vi "SwapInstanceVIUnusedName2 40.vi"(6 "Bindata & descr in":T1, 7 "type":i16, 8 "error in (no error)":errorcluster, 9 "dims":u8=3 min=1 max=3, 11 "kwarg_name":string="testarg") -> (0 "error out":errorcluster, 1 "Array 3D":i16[][][](array[numeric]), 2 "Array 2D":i16[][](array[numeric]), 3 "Array 1D":i16[](array[numeric]), 4 "Bindata & descr out":T1, 5 "bindata":u8[](array[numeric]))   [LabVIEW 2018]
uses:
  Bindata&description.ctl
  Bindata description.ctl
  b16ececd-46f8-40b8-a446-7cfb86b2ab33.vi
  2e3b4c87-8736-4d5a-badb-c1f06a639308.vi
  c6e5ccd4-8fd0-42b7-a10f-f76efdbd56f8.vi
  4bd48677-245d-4e5f-868b-8f16d0eed5f9.vi
  2e3b4c87-8736-4d5a-badb-c1f06a639308.vi/0d828339-51f4-44c0-8bf4-a630556f2914.vi
  c6e5ccd4-8fd0-42b7-a10f-f76efdbd56f8.vi/48ec535c-94cf-46ee-ad69-877121677c8d.vi
  4bd48677-245d-4e5f-868b-8f16d0eed5f9.vi/cfc365a5-ff30-4df4-9512-66e4ce510117.vi
  2e3b4c87-8736-4d5a-badb-c1f06a639308.vi/0d828339-51f4-44c0-8bf4-a630556f2914.vi/dacc63a1-9bba-4eb3-b6b7-9f46c6cc7eba.vi
  c6e5ccd4-8fd0-42b7-a10f-f76efdbd56f8.vi/48ec535c-94cf-46ee-ad69-877121677c8d.vi/1c39fd07-564b-4c6f-bc60-59ab712499e7.vi
  4bd48677-245d-4e5f-868b-8f16d0eed5f9.vi/cfc365a5-ff30-4df4-9512-66e4ce510117.vi/5adf2ae5-6315-4e22-a618-f07e80211284.vi
  2e3b4c87-8736-4d5a-badb-c1f06a639308.vi/0d828339-51f4-44c0-8bf4-a630556f2914.vi/dacc63a1-9bba-4eb3-b6b7-9f46c6cc7eba.vi/dc3be9b1-6013-443b-b0cf-b3c472992a41.vi
  c6e5ccd4-8fd0-42b7-a10f-f76efdbd56f8.vi/48ec535c-94cf-46ee-ad69-877121677c8d.vi/1c39fd07-564b-4c6f-bc60-59ab712499e7.vi/3418dce5-cf0d-4204-8015-2e708795db54.vi
  4bd48677-245d-4e5f-868b-8f16d0eed5f9.vi/cfc365a5-ff30-4df4-9512-66e4ce510117.vi/5adf2ae5-6315-4e22-a618-f07e80211284.vi/54620dc9-9476-40af-bea6-8759de6f1d7f.vi
  check ID validity.vi
  LV-Julia_ZMQ-Roundtrip_lib.lvlib
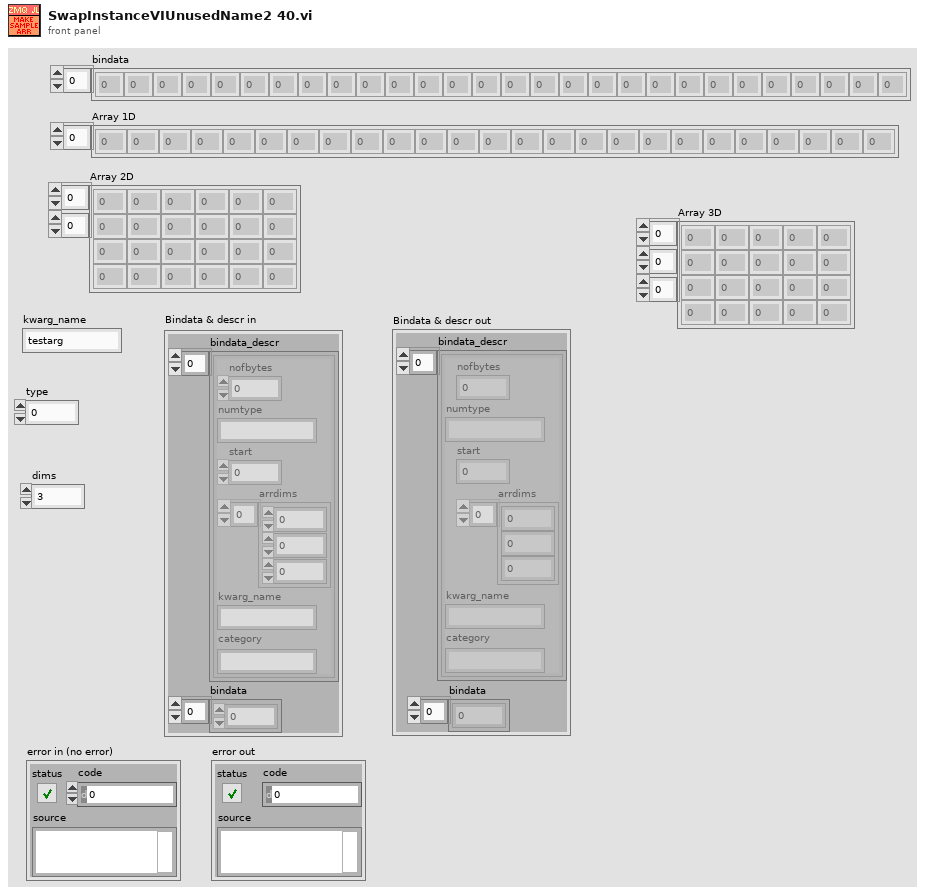
[diagram p1: front panel]
types:
  T1 = typedef "Bindata&description.ctl" = cluster{"bindata_descr":T2[], "bindata":u8[]}
  T2 = typedef "LV-Julia_ZMQ-Roundtrip_lib.lvlib/Bindata description.ctl" = cluster{"nofbytes":i32, "numtype":string, "start":i32, "arrdims":i32[], "kwarg_name":string, "category":string}
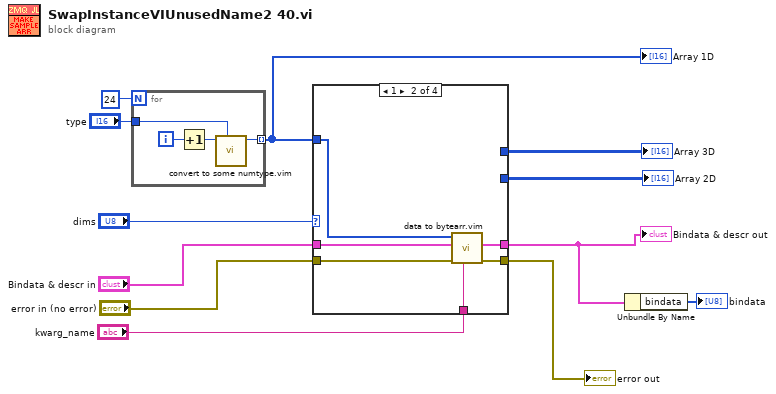
[diagram p0: block diagram]
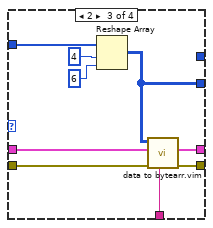
[diagram p3: hidden frame]
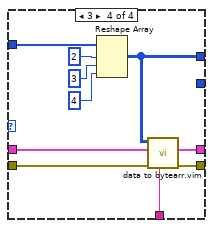
[diagram p4: hidden frame]
diagram:
  n1 = for {
    N: 24 -> [_]
    tunnel: [w14] -> w11 mode=indexing
    tunnel: "type" -> [w13]
    i -> [w16]
    n2 = Increment(x=w16) -> (x+1=w15:i32)
    n3 = call "convert to some numtype.vim"("type"=w13, "Numeric in"=w15) -> ("Numeric out"=w14:i16)  [unwired: 9 in]
  }
  "Array 1D" <- w11
  n4 = case shown="1" "dims" {
    tunnel: [_ _ _ w42] -> w12
    tunnel: w11 -> [_ w23 w30 w38]
    tunnel: "kwarg_name" -> [_ w22 w29 w37]
    tunnel: "error in (no error)" -> [w17 w21 w28 w36]
    tunnel: [w17 w20 w27 w35] -> w5
    tunnel: [_ w19 w26 w34] -> w2
    tunnel: [_ _ w25 _] -> w4
    tunnel: "Bindata & descr in" -> [_ w18 w24 w33]
    frame 0, Default {
    }
    frame 1 {
      n5 = call "data to bytearr.vim"("kwarg_name"=w22, "error in (no error)"=w21, "Bindata & descr in"=w18, "data in"=w23) -> ("error out"=w20:errorcluster, "Bindata & descr out"=w19:T1)  [unwired: 5 in, 1 out]
    }
    frame 2 {
      n6 = Reshape Array(w30, 4 ("dimension size"), 6 ("dimension size")) -> (w25:i16[][])
      n7 = call "data to bytearr.vim"("kwarg_name"=w29, "error in (no error)"=w28, "Bindata & descr in"=w24, "data in"=w25) -> ("error out"=w27:errorcluster, "Bindata & descr out"=w26:T1)  [unwired: 5 in, 1 out]
    }
    frame 3 {
      n8 = Reshape Array(w38, 2 ("dimension size"), 3 ("dimension size"), 4 ("dimension size")) -> (w42:i16[][][])
      n9 = call "data to bytearr.vim"("kwarg_name"=w37, "error in (no error)"=w36, "Bindata & descr in"=w33, "data in"=w42) -> ("error out"=w35:errorcluster, "Bindata & descr out"=w34:T1)  [unwired: 5 in, 1 out]
    }
  }
  "Array 3D" <- w12
  "Bindata & descr out" <- w2
  "error out" <- w5
  "Array 2D" <- w4
  n10 = Unbundle By Name(w2) -> ("bindata"=→"bindata":u8[])
